vi "TRC_Query.vi"(0 "System no.":i32=1 min=1 max=4 step=1, 5 "error in":errorcluster) -> (14 "Number of relays":i32, 19 "error out":errorcluster)   [LabVIEW 2020]
doc: "Returns the number of relays available in the controller (one relay board supports 8 relays)."
panel:
  # "Returns the number of relays available in the controller (one \nrelay board supports 8 relays)."
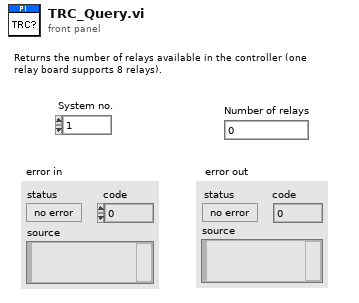
[diagram p1: front panel]
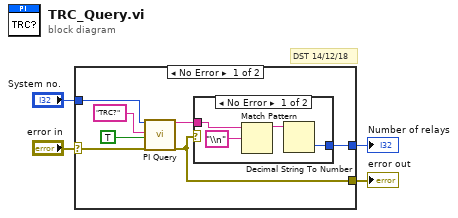
[diagram p0: block diagram]
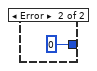
[diagram p2: hidden frame]
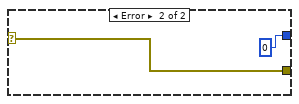
[diagram p3: hidden frame]
diagram:
  # "DST 14/12/18"
  n1 = case shown="No Error" "error in" {
    selector: "error in" -> [w7 w18]
    tunnel: [w11 0] -> w4
    tunnel: "System no." -> [w9 _]
    tunnel: [w5 w18] -> w2
    frame No Error {
      n2 = call "PI Query.vi"("System no."=w9, "String to send"="TRC?", "Attach termination char.?"=TRUE ("Attach Linefeed?"), "error in"=w7) -> ("String read"=w6:string, "error out"=w5:errorcluster)  [unwired: 3 in, 11 out]
      n3 = case shown="No Error" w5 {
        tunnel: w6 -> [w14 _]
        tunnel: [w15 0] -> w11
        frame No Error {
          n4 = Match Pattern(string=w14, regular expression="\\n") -> (before substring=w12:string)  [unwired: 4 out]
          n5 = Decimal String To Number(string=w12) -> (number=w15:i32)  [unwired: 3 out]
        }
        frame Error {
        }
      }
    }
    frame Error {
    }
  }
  "error out" <- w2
  "Number of relays" <- w4
